vi "Get acq type.vi"(11 "Task in":refnum<k21>) -> (3 "Acq type":T1)   [LabVIEW 2020, in "NI DAQ Aug 25.lvlib"]
uses:
  NI DAQ Aug 25.lvlib
  Acquisition type--typedef.ctl
  <resource>/objmgr/daqmx.rc
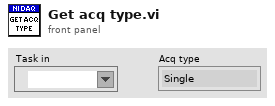
[diagram p1: front panel]
types:
  T1 = typedef "NI DAQ Aug 25.lvlib/Acquisition type--typedef.ctl" = enum16{"Single", "Multiple"}
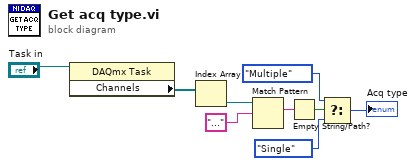
[diagram p0: block diagram]
diagram:
  n1 = property class="DAQmx Task"(reference="Task in") -> ("Channels"=w3:refnum<k21>[])  [unwired: 1 in, 2 out]
  n2 = Index Array(array=w3) -> (element=w4:refnum<k21>)  [unwired: 1 in]
  n3 = Match Pattern(string=w4, regular expression="...") -> (match substring=w7:string)  [unwired: 1 in, 3 out]
  n4 = Empty String/Path?(string/path=w7) -> (empty?=w6:bool)
  n5 = Select(t=Acquisition_type--typedef."Multiple" ("Acq type"), s=w6, f=Acquisition_type--typedef."Single" ("Acq type")) -> (s? t:f=→"Acq type":T1)
